vi "Load saved scan settings.vi"() -> (0 "Scan settings array":T1[](array[typedef]), 3 "Scan settings name array":string[](array[string]), 4 "Settings folder path":path)   [LabVIEW 2011]
uses:
  <vilib>/Utility/file.llb/Read From Spreadsheet File (string).vi
  TypeDefs/Settings Boolean.ctl
  TypeDefs/Scan settings.ctl
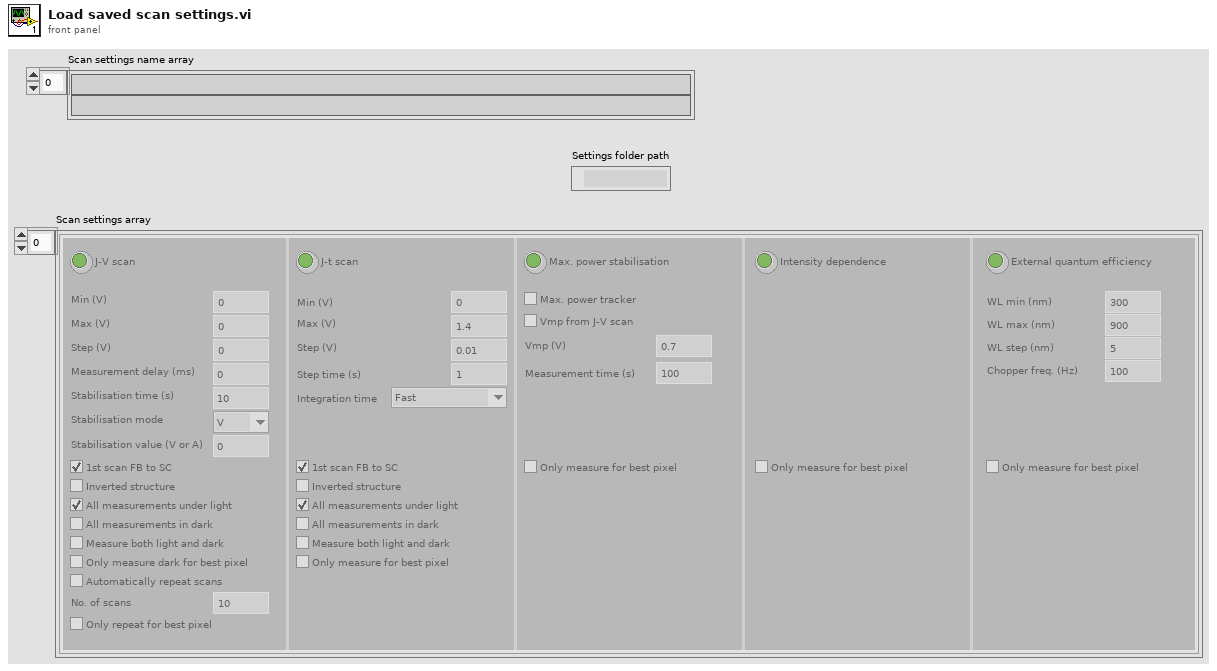
[diagram p1: front panel]
types:
  T1 = typedef "Scan settings.ctl" = cluster{"J-V scan":T2, "Min (V)":dbl, "Max (V)":dbl, "Step (V)":dbl, "Measurement delay (ms)":dbl, "Stabilisation time (s)":dbl, "Stabilisation mode":enum16{"V", "I"}, "Stabilisation value (V or A) ":dbl, "1st scan FB-SC":bool, "Inverted structure":bool, "All measurements under light":bool, "Dark J-V only":bool, "Light and dark measurements":bool, "Only measure in dark for best pixel":bool, "Repeat each scan 10 times":bool, "J-t scan":bool, "J-t Min (V)":dbl, "J-t Max (V)":dbl, "J-t Step (V)":dbl, "Step time (s)":dbl, "Integration time":enum16{"Fast", "Normal", "High Accuracy"}, "J-t 1st scan FB-SC":bool, "J-t Inverted structure":bool, "J-t All measurements under light":bool, "J-t Dark only":bool, "J-t Light and dark":bool, "J-t best pixel only":bool, "Max. power stabilisation":bool, "Max power tracking":bool, "Vmp from J-V scan":bool, "Vmp (V)":dbl, "Measurement time (s)":dbl, "Max power best pixel only":bool, "Intensity dependence":bool, "P dep best pixel only":bool, "External quantum efficiency":bool, "EQE best pixel only":bool, "WL min (nm)":dbl, "WL max (nm)":dbl, "WL step (nm)":dbl, "Chopper freq. (Hz)":dbl, "No. of scans":dbl, "Only repeat for best pixel":bool}
  T2 = typedef "Settings Boolean.ctl" = bool
  T3 = cluster{"J-V scan":bool, "J-t scan":bool, "Min (V)":dbl, "Max (V)":dbl, "Step (V)":dbl, "Measurement delay (ms)":dbl, "1st scan FB-SC":bool, "Inverted structure":bool, "Stabilisation time (s)":dbl, "Stabilisation mode":enum16{"V", "I"}, "Stabilisation value (V or A) ":dbl, "Step time (s)":dbl, "Integration time":enum16{"Fast", "Normal", "High Accuracy"}, "Repeat each scan 10 times":bool, "Dark J-V only":bool, "Light and dark measurements":bool, "Only measure in dark for best pixel":bool, "All measurements under light":bool}
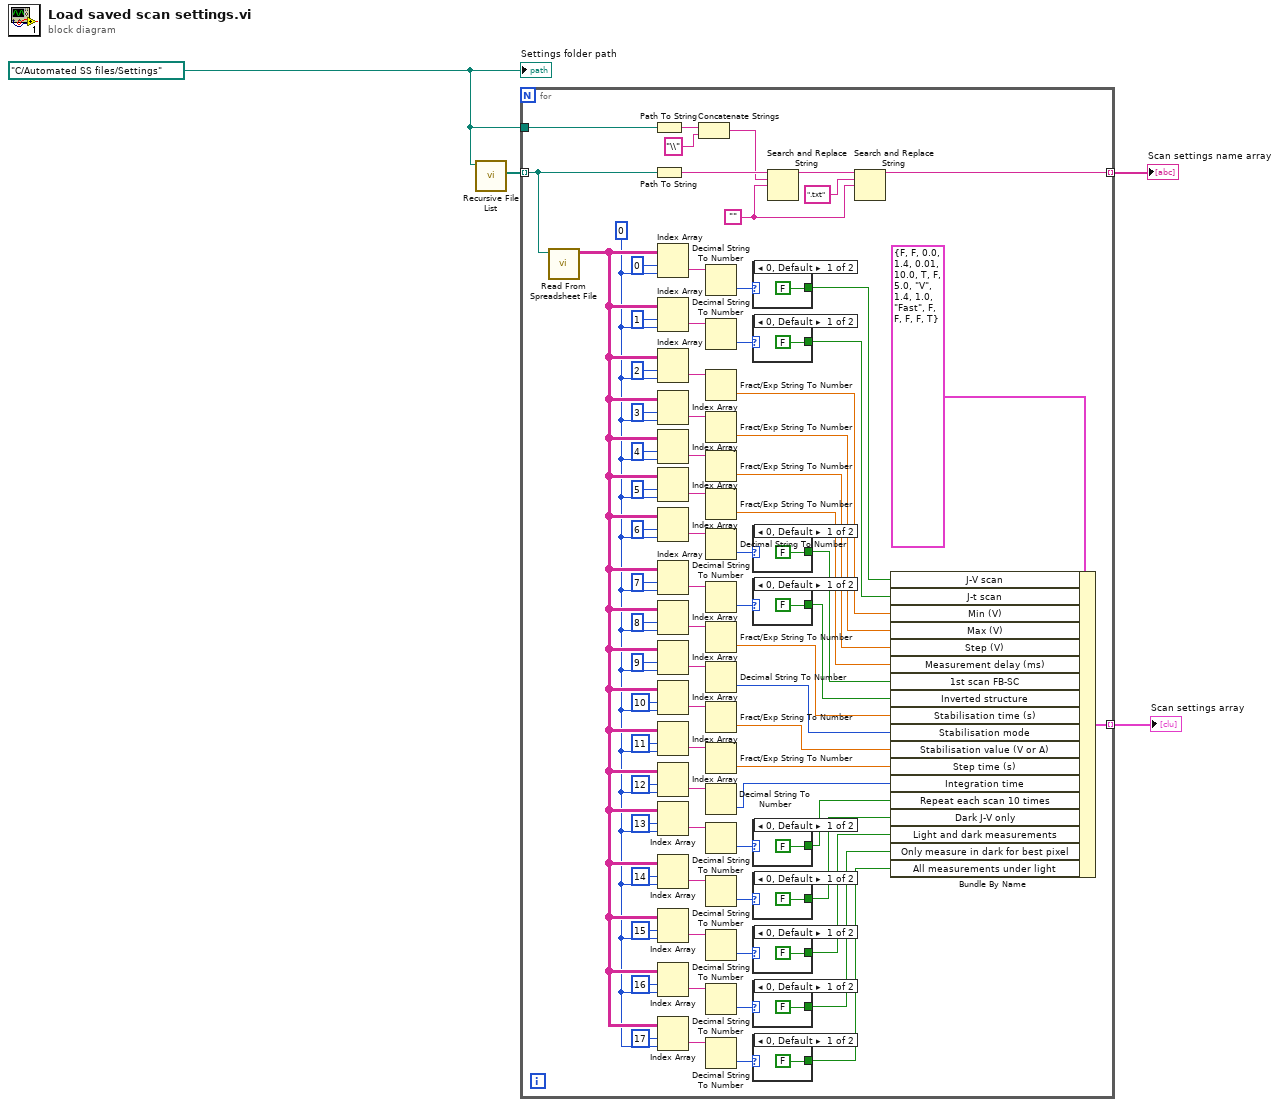
[diagram p0: block diagram]
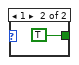
[diagram p2: hidden frame]
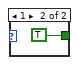
[diagram p3: hidden frame]
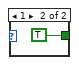
[diagram p4: hidden frame]
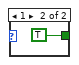
[diagram p5: hidden frame]
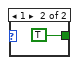
[diagram p6: hidden frame]
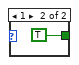
[diagram p7: hidden frame]
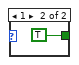
[diagram p8: hidden frame]
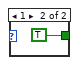
[diagram p9: hidden frame]
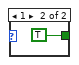
[diagram p10: hidden frame]
diagram:
  w1 = path "C:/Automated SS files/Settings"
  n1 = call <vilib>:"Recursive File List.vi"("Folder Path"=w1) -> ("All Files in Dir"=w4:path[])  [unwired: 6 in, 4 out]
  n2 = for {
    tunnel: w4 -> [w15] mode=indexing
    tunnel: [w13] -> w3 mode=indexing
    tunnel: [w12] -> w2 mode=indexing
    tunnel: w1 -> [w11]
    w9 = ""
    w80 = 0
    n3 = call-poly <vilib>:"Read From Spreadsheet File.vi"("file path (dialog if empty)"=w15) -> ("all rows"=w81:string[][])  [unwired: 6 in, 4 out]
    n4 = Path To String(path=w11) -> (string=w7:string)
    n5 = Path To String(path=w15) -> (string=w10:string)
    n6 = Index Array(array=w81, index (row)=0, index (col)=w80) -> (element=w60:string)
    n7 = Index Array(array=w81, index (row)=1, index (col)=w80) -> (element=w58:string)
    n8 = Index Array(array=w81, index (row)=2, index (col)=w80) -> (element=w57:string)
    n9 = Index Array(array=w81, index (row)=3, index (col)=w80) -> (element=w56:string)
    n10 = Index Array(array=w81, index (row)=4, index (col)=w80) -> (element=w55:string)
    n11 = Index Array(array=w81, index (row)=5, index (col)=w80) -> (element=w54:string)
    n12 = Index Array(array=w81, index (row)=6, index (col)=w80) -> (element=w51:string)
    n13 = Index Array(array=w81, index (row)=7, index (col)=w80) -> (element=w50:string)
    n14 = Index Array(array=w81, index (row)=8, index (col)=w80) -> (element=w49:string)
    n15 = Index Array(array=w81, index (row)=9, index (col)=w80) -> (element=w48:string)
    n16 = Index Array(array=w81, index (row)=10, index (col)=w80) -> (element=w47:string)
    n17 = Index Array(array=w81, index (row)=11, index (col)=w80) -> (element=w46:string)
    n18 = Index Array(array=w81, index (row)=12, index (col)=w80) -> (element=w45:string)
    n19 = Index Array(array=w81, index (row)=13, index (col)=w80) -> (element=w39:string)
    n20 = Index Array(array=w81, index (row)=14, index (col)=w80) -> (element=w38:string)
    n21 = Index Array(array=w81, index (row)=15, index (col)=w80) -> (element=w37:string)
    n22 = Index Array(array=w81, index (row)=16, index (col)=w80) -> (element=w36:string)
    n23 = Index Array(array=w81, index (row)=17, index (col)=w80) -> (element=w35:string)
    n24 = Concatenate Strings(w7, "\\") -> (w5:string)
    n25 = Decimal String To Number(string=w60) -> (number=w61:i32)  [unwired: 2 in, 1 out]
    n26 = Decimal String To Number(string=w58) -> (number=w59:i32)  [unwired: 2 in, 1 out]
    n27 = Fract/Exp String To Number(string=w57) -> (number=w31:dbl)  [unwired: 3 in, 1 out]
    n28 = Fract/Exp String To Number(string=w56) -> (number=w30:dbl)  [unwired: 3 in, 1 out]
    n29 = Fract/Exp String To Number(string=w55) -> (number=w28:dbl)  [unwired: 3 in, 1 out]
    n30 = Fract/Exp String To Number(string=w54) -> (number=w27:dbl)  [unwired: 3 in, 1 out]
    n31 = Decimal String To Number(string=w51) -> (number=w53:i32)  [unwired: 2 in, 1 out]
    n32 = Decimal String To Number(string=w50) -> (number=w52:i32)  [unwired: 2 in, 1 out]
    n33 = Fract/Exp String To Number(string=w49) -> (number=w25:dbl)  [unwired: 3 in, 1 out]
    n34 = Decimal String To Number(string=w48) -> (number=w24:i32)  [unwired: 2 in, 1 out]
    n35 = Fract/Exp String To Number(string=w47) -> (number=w23:dbl)  [unwired: 3 in, 1 out]
    n36 = Fract/Exp String To Number(string=w46) -> (number=w22:dbl)  [unwired: 3 in, 1 out]
    n37 = Decimal String To Number(string=w45) -> (number=w21:i32)  [unwired: 2 in, 1 out]
    n38 = Decimal String To Number(string=w39) -> (number=w44:i32)  [unwired: 2 in, 1 out]
    n39 = Decimal String To Number(string=w38) -> (number=w43:i32)  [unwired: 2 in, 1 out]
    n40 = Decimal String To Number(string=w37) -> (number=w41:i32)  [unwired: 2 in, 1 out]
    n41 = Decimal String To Number(string=w36) -> (number=w42:i32)  [unwired: 2 in, 1 out]
    n42 = Decimal String To Number(string=w35) -> (number=w40:i32)  [unwired: 2 in, 1 out]
    n43 = case shown="0, Default" w61 {
      tunnel: [FALSE TRUE] -> w34
      frame 0, Default {
      }
      frame 1 {
      }
    }
    n44 = case shown="0, Default" w59 {
      tunnel: [FALSE TRUE] -> w32
      frame 0, Default {
      }
      frame 1 {
      }
    }
    n45 = case shown="0, Default" w53 {
      tunnel: [FALSE TRUE] -> w29
      frame 0, Default {
      }
      frame 1 {
      }
    }
    n46 = case shown="0, Default" w52 {
      tunnel: [FALSE TRUE] -> w26
      frame 0, Default {
      }
      frame 1 {
      }
    }
    n47 = case shown="0, Default" w44 {
      tunnel: [FALSE TRUE] -> w20
      frame 0, Default {
      }
      frame 1 {
      }
    }
    n48 = case shown="0, Default" w43 {
      tunnel: [FALSE TRUE] -> w19
      frame 0, Default {
      }
      frame 1 {
      }
    }
    n49 = case shown="0, Default" w41 {
      tunnel: [FALSE TRUE] -> w18
      frame 0, Default {
      }
      frame 1 {
      }
    }
    n50 = case shown="0, Default" w42 {
      tunnel: [FALSE TRUE] -> w17
      frame 0, Default {
      }
      frame 1 {
      }
    }
    n51 = case shown="0, Default" w40 {
      tunnel: [FALSE TRUE] -> w16
      frame 0, Default {
      }
      frame 1 {
      }
    }
    n52 = Search and Replace String(input string=w10, search string=w5, replace string=w9) -> (result string=w8:string)  [unwired: 5 in, 3 out]
    n53 = Search and Replace String(input string=w8, search string=".txt", replace string=w9) -> (result string=w12:string)  [unwired: 5 in, 3 out]
    n54 = Bundle By Name(cluster=T3 {"J-V scan"=FALSE, "J-t scan"=FALSE, "Min (V)"=0.0, "Max (V)"=1.4, "Step (V)"=0.01, "Measurement delay (ms)"=10.0, "1st scan FB-SC"=TRUE, "Inverted structure"=FALSE, "Stabilisation time (s)"=5.0, "Stabilisation mode"=enum."V", "Stabilisation value (V or A) "=1.4, "Step time (s)"=1.0, "Integration time"=enum."Fast", "Repeat each scan 10 times"=FALSE, "Dark J-V only"=FALSE, "Light and dark measurements"=FALSE, "Only measure in dark for best pixel"=FALSE, "All measurements under light"=TRUE} ("New scan settings 2"), "J-V scan"=w34, "J-t scan"=w32, "Min (V)"=w31, "Max (V)"=w30, "Step (V)"=w28, "Measurement delay (ms)"=w27, "1st scan FB-SC"=w29, "Inverted structure"=w26, "Stabilisation time (s)"=w25, "Stabilisation mode"=w24, "Stabilisation value (V or A)"=w23, "Step time (s)"=w22, "Integration time"=w21, "Repeat each scan 10 times"=w20, "Dark J-V only"=w19, "Light and dark measurements"=w18, "Only measure in dark for best pixel"=w17, "All measurements under light"=w16) -> (w13:T3)
  }
  "Scan settings array" <- w3
  "Scan settings name array" <- w2
  "Settings folder path" <- w1
